vi "Write Observe Data Msg Return Info.vi"(8 "Return Priority (Normal)":T1=enum."Normal", 9 "Datum Name":string, 10 "Message Enqueuer in":refnum<class "Message Enqueuer.lvclass">, 11 "Observe Data Msg In":refnum<class "Observe Data Msg.lvclass">) -> (3 "Observe Data Msg Out":refnum<class "Observe Data Msg.lvclass">)   [LabVIEW 2020, in "IObserver.lvlib" / "Observe Data Msg.lvclass"]
doc: "<License>\nCopyright © 2017 Composed Systems, LLC | All rights reserved\nwww.composed.io\n\nAuthor: Ethan Stern <ethan.stern@composed.io>\n\nThis software is provided \"AS IS\" WITHOUT WARRANTIES, either express or implied, AND IS FOR EDUCATIONAL PURPOSES ONLY.\n</License>"
uses:
  Observe Data Msg.lvclass
  <vilib>/ActorFramework/Message Enqueuer/Message Enqueuer.lvclass
  <vilib>/ActorFramework/Message Enqueuer/Message Priority.ctl
  Observe Data Msg.lvclass/Observe Data Msg.ctl
  composed-af-messages/Source/RoundTripMessage/RoundTripMessage.lvclass/RoundTripMessage.ctl
  composed-af-messages/Source/RoundTripMessage/RoundTripMessage.lvclass
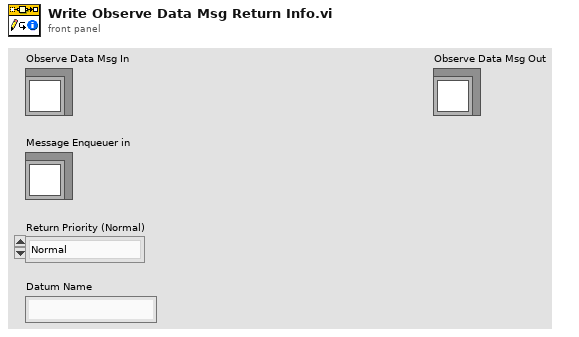
[diagram p1: front panel]
types:
  T1 = typedef "Actor Framework.lvlib/Message Enqueuer.lvclass/Message Priority.ctl" = enum16{"Low", "Normal", "High"}
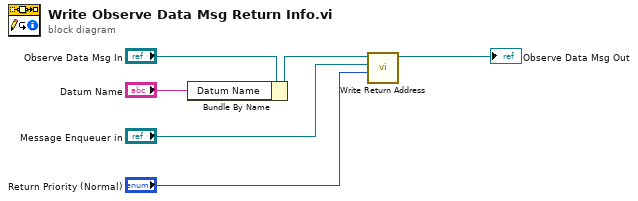
[diagram p0: block diagram]
diagram:
  n1 = Bundle By Name(cluster="Observe Data Msg In", "Datum Name"="Datum Name") -> (w2:refnum<class "Observe Data Msg.lvclass">)
  n2 = call "Write Return Address.vi"("Return Priority (Normal)"="Return Priority (Normal)", "Return Enqueuer"="Message Enqueuer in", "RoundTripMessage In"=w2) -> ("RoundTripMessage Out"=→"Observe Data Msg Out":refnum<class "Observe Data Msg.lvclass">)  [unwired: 8 in]
